vi "UpdateSpkCycle.vi"(7 "LabVIEW Web Service Request":refnum<class "Web Request.lvclass">, 9 "Length":i16, 10 "Period":i16, 11 "Cycle":u8) -> ()   [LabVIEW 2014]
uses:
  <vilib>/wsapi/Web Request.lvclass
  Instr Actor/Messages/Speaker Cycle MSG/Spk Cycle MSG.lvclass
  Controller/Controls/Enqueuer Enum.ctl
  Instr Actor/Messages/Speaker Cycle MSG/Spk Cycle MSG.lvclass/Spk Cycle MSG.ctl
  Instr Actor/Messages/Speaker Cycle MSG/Write Cycle_.vi
  Instr Actor/Messages/Speaker Cycle MSG/Write Length.vi
  Instr Actor/Messages/Speaker Cycle MSG/Write Period.vi
  Controller/Controller.lvclass
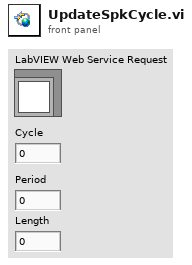
[diagram p1: front panel]
types:
  T1 = typedef "Enqueuer Enum.ctl" = enum8{"PAS", "CRDS", "File"}
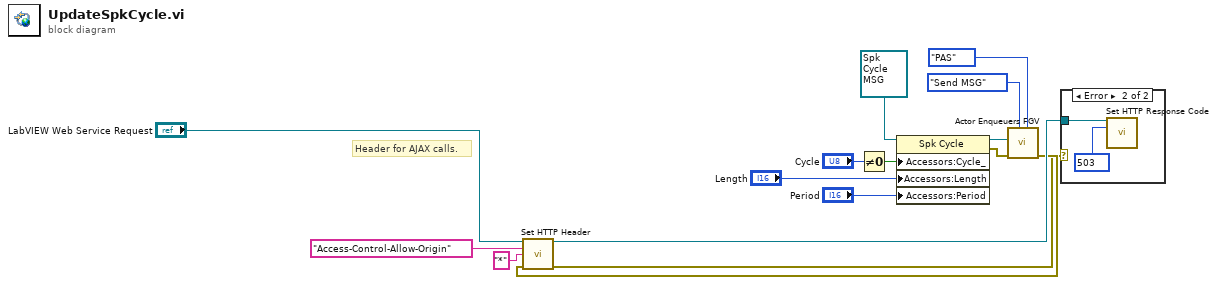
[diagram p0: block diagram]
diagram:
  # "Header for AJAX calls."
  n1 = Not Equal To 0?(x="Cycle") -> (x != 0?=w13:bool)
  n2 = property class="Spk Cycle"(reference=refnum<class "Spk Cycle MSG.lvclass"> refnum ("Instrument Lib:Spk Cycle MSG.lvclass"), "Accessors:Cycle_"=w13, "Accessors:Length"="Length", "Accessors:Period"="Period") -> (reference out=w10:refnum<class "Spk Cycle MSG.lvclass">, error out=w9:errorcluster)  [unwired: 1 in]
  n3 = call "Actor Enqueuers FGV.vi"("Enqueuer"=Enqueuer_Enum."PAS", "State"=enum16{"Store", "Send MSG"}."Send MSG", "error in"=w9, "MSG"=w10) -> ("error out"=w2:errorcluster)  [unwired: 7 in]
  n4 = call <vilib>:"Set HTTP Header.vi"("LabVIEW Web Service Request"="LabVIEW Web Service Request", "header"="Access-Control-Allow-Origin", "header value"="*", "error in (no error)"=w2) -> ("LabVIEW Web Service Request out"=w4:refnum<class "Web Request.lvclass">, "error out"=w1:errorcluster)  [unwired: 10 in]
  n5 = case shown="Error" w1 {
    tunnel: w4 -> [_ w16]
    frame No Error {
    }
    frame Error {
      w17 = 503 items=["100"=100, "101"=101, "200"=200, "201"=201, "202"=202, "203"=203, "204"=204, "205"=205, "206"=206, "300"=300, "301"=301, "302"=302, "303"=303, "304"=304, "305"=305, "306"=306, "307"=307, "400"=400, "401"=401, "402"=402, "403"=403, "404"=404, "405"=405, "406"=406, "407"=407, "408"=408, "409"=409, "410"=410, "411"=411, "412"=412, "413"=413, "414"=414, "415"=415, "416"=416, "417"=417, "500"=500, "501"=501, "502"=502, "503"=503, "504"=504, "505"=505] ("response code (200)")
      n6 = call <vilib>:"Set HTTP Response Code.vi"("LabVIEW Web Service Request"=w16, "response code (200)"=w17) -> ()  [unwired: 12 in, 2 out]
    }
  }
